vi "REWORK_create_queues.vi"(8 "error_in":errorcluster, 11 "all_config_info_in":T1={"main_ini_file"={"SQL Driver"="", "SQL Server"="", "SQL Database"="", "SQL UID"="", "User table"="", "default language"="", "SCANNER COM port"=0, "SCANNER Baud rate"=0, "SCANNER Data bits"=0, "SCANNER Pairity"=enum."None", "SCANNER Stop bits"=10, "SCANNER Flow control"=0, "SCANNER Termination char"=0, "ST 140 name"="", "ST 140 listener IP"="", "ST 140 listener port"=0, "logout timeout [ms]"=0}, "SQL Password"="", "queue_refnums"={"MAIN_queue"=refnum, "SCANNER_queue"=refnum, "SCANNER_data"=refnum}} {"main_ini_file"."SCANNER Flow control" items=["None"=0, "XON/XOFF"=1, "RTS/CTS"=2, "DTR/DSR"=4]; "main_ini_file"."SCANNER Stop bits" items=["1.0"=10, "1.5"=15, "2.0"=20]}) -> (0 "error_out":errorcluster, 3 "all_config_info_out":T1={"main_ini_file"={"SQL Driver"="", "SQL Server"="", "SQL Database"="", "SQL UID"="", "User table"="", "default language"="", "SCANNER COM port"=0, "SCANNER Baud rate"=0, "SCANNER Data bits"=0, "SCANNER Pairity"=enum."None", "SCANNER Stop bits"=10, "SCANNER Flow control"=0, "SCANNER Termination char"=0, "ST 140 name"="", "ST 140 listener IP"="", "ST 140 listener port"=0, "logout timeout [ms]"=0}, "SQL Password"="", "queue_refnums"={"MAIN_queue"=refnum, "SCANNER_queue"=refnum, "SCANNER_data"=refnum}} {"main_ini_file"."SCANNER Flow control" items=["None"=0, "XON/XOFF"=1, "RTS/CTS"=2, "DTR/DSR"=4]; "main_ini_file"."SCANNER Stop bits" items=["1.0"=10, "1.5"=15, "2.0"=20]})   [LabVIEW 2019]
uses:
  ini/typedef/REWORK_all_config_info.ctl
  ini/typedef/REWORK_main_ini_file.ctl
  typedef/REWORK_queue_refnums.ctl
  typedef/REWORK_MAIN_queue_element.ctl
  MAIN/REWORK_MAIN_sequence_state.ctl
  typedef/REWORK_SCANNER_queue_element.ctl
  SCANNER/REWORK_SCANNER_sequence_state.ctl
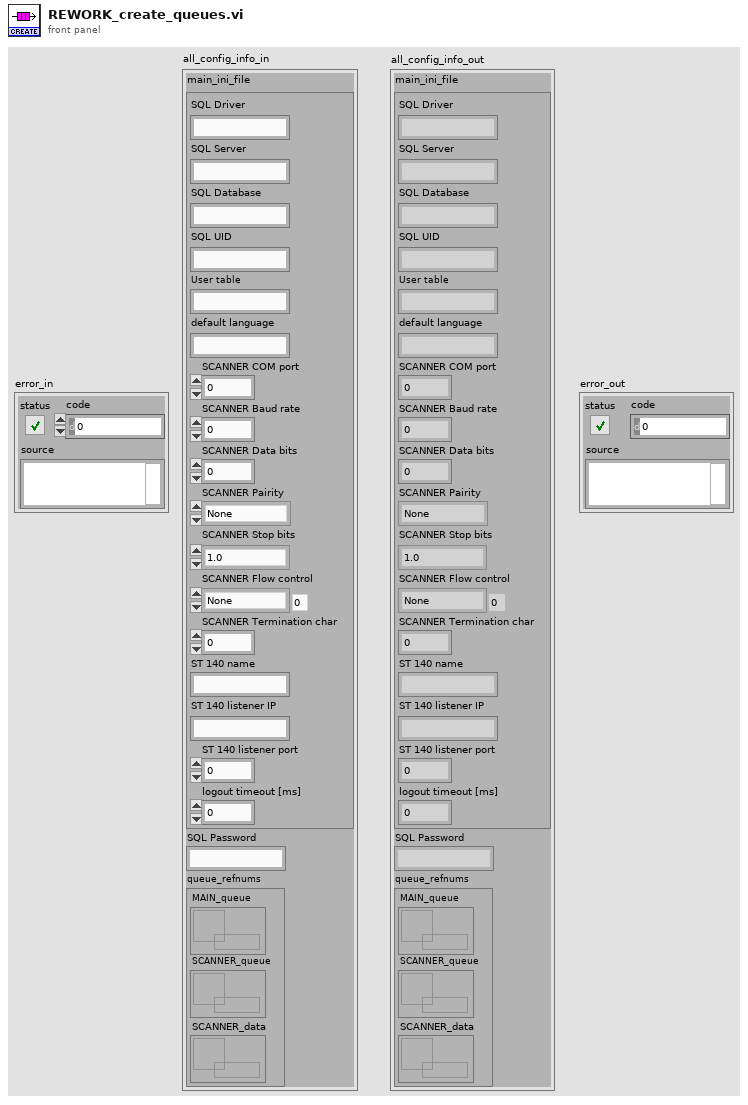
[diagram p1: front panel]
types:
  T1 = typedef "REWORK_all_config_info.ctl" = cluster{"main_ini_file":T2, "SQL Password":string, "queue_refnums":T3}
  T2 = typedef "REWORK_main_ini_file.ctl" = cluster{"SQL Driver":string, "SQL Server":string, "SQL Database":string, "SQL UID":string, "User table":string, "default language":string, "SCANNER COM port":u16, "SCANNER Baud rate":u32, "SCANNER Data bits":u16, "SCANNER Pairity":enum16{"None", "Odd", "Even", "Mark", "Space"}, "SCANNER Stop bits":u16, "SCANNER Flow control":u16, "SCANNER Termination char":u8, "ST 140 name":string, "ST 140 listener IP":string, "ST 140 listener port":u16, "logout timeout [ms]":i32}
  T3 = typedef "REWORK_queue_refnums.ctl" = cluster{"MAIN_queue":refnum<queue>, "SCANNER_queue":refnum<queue>, "SCANNER_data":refnum<queue>}
  T4 = typedef "REWORK_SCANNER_queue_element.ctl" = cluster{"state":T5, "variable":variant}
  T5 = typedef "REWORK_SCANNER_sequence_state.ctl" = enum16{"initialize", "get_next_state", "read", "cancel_read", "error", "stop"}
  T6 = typedef "REWORK_MAIN_queue_element.ctl" = cluster{"state":T7, "variable":variant}
  T7 = typedef "REWORK_MAIN_sequence_state.ctl" = enum16{"initialize", "get_next_state", "parse_TCP", "send_TCP_response", "REWORK_commit", "USER_login", "USER_logout", "clear_gear_data", "error", "stop"}
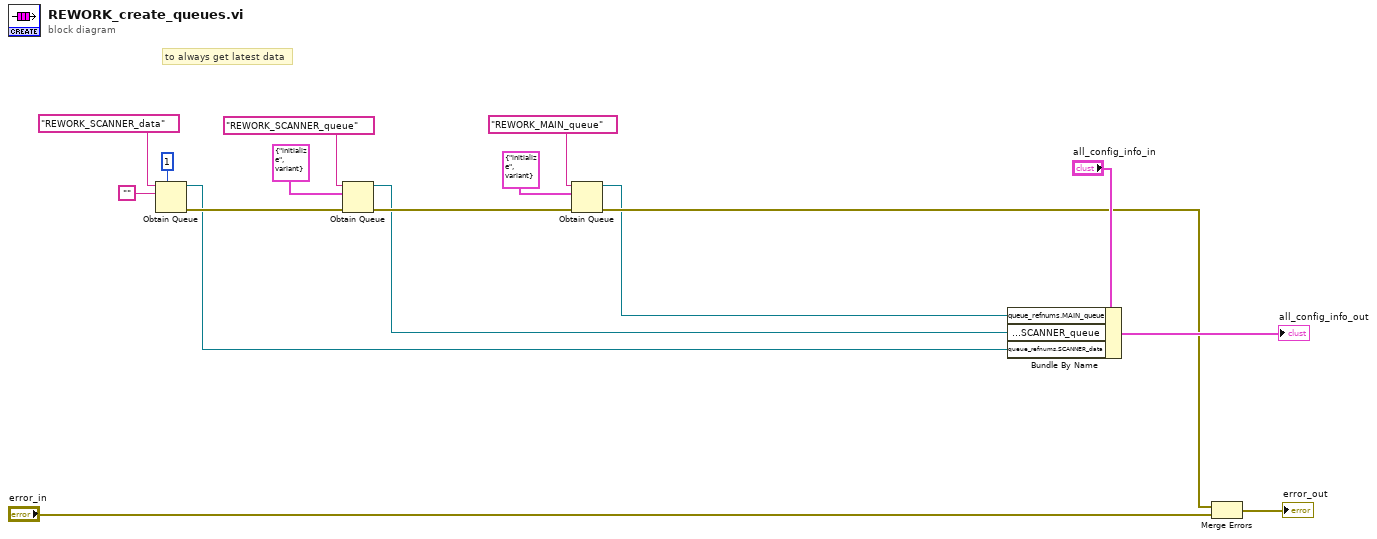
[diagram p0: block diagram]
diagram:
  # "to always get latest data"
  n1 = Obtain Queue(max queue size (-1, unlimited)=1, name (unnamed)="REWORK_SCANNER_data", element data type="") -> (queue out=w4:refnum<queue>, error out=w7:errorcluster)  [unwired: 2 in, 1 out]
  n2 = Obtain Queue(name (unnamed)="REWORK_SCANNER_queue", element data type=T4 {"state"=enum."initialize", "variable"=variant} ("SCANNER_queue_element"), error in (no error)=w7) -> (queue out=w1:refnum<queue>, error out=w10:errorcluster)  [unwired: 2 in, 1 out]
  n3 = Obtain Queue(name (unnamed)="REWORK_MAIN_queue", element data type=T6 {"state"=enum."initialize", "variable"=variant} ("MANUAL_SQL_CON_queue_element"), error in (no error)=w10) -> (queue out=w2:refnum<queue>, error out=w11:errorcluster)  [unwired: 2 in, 1 out]
  n4 = Bundle By Name(cluster="all_config_info_in", "queue_refnums.MAIN_queue"=w2, "queue_refnums.SCANNER_queue"=w1, "queue_refnums.SCANNER_data"=w4) -> (→"all_config_info_out":T1)
  n5 = Merge Errors(w11, "error_in") -> (→"error_out":errorcluster)
